vi "Convert Parameter string to 2D array.vi"(8 "Error In":errorcluster, 11 "Parameter string IN (without paranthesis)":string) -> (0 "Error Out":errorcluster, 1 "offset of last detected comma (0 if none)":i32, 2 "Number of commas":i32, 3 "Params table OUT":string[][](array[string]))   [LabVIEW 2012]
doc: "SciScan 1.2 160622"
uses:
  <vilib>/regexp/Match Regular Expression.xnode
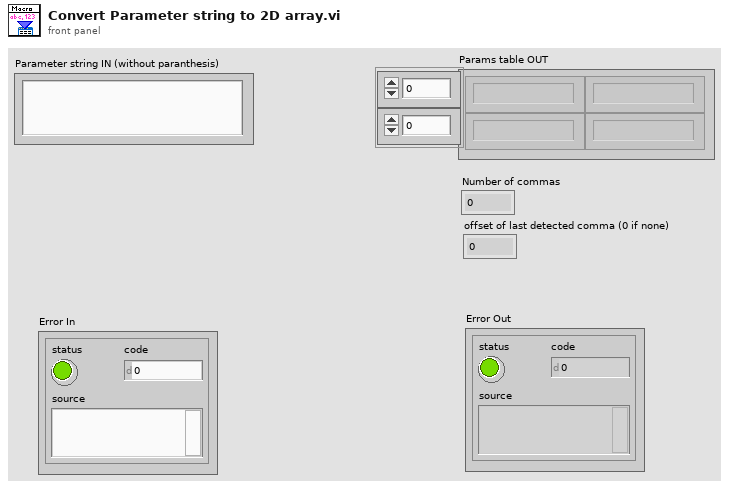
[diagram p1: front panel]
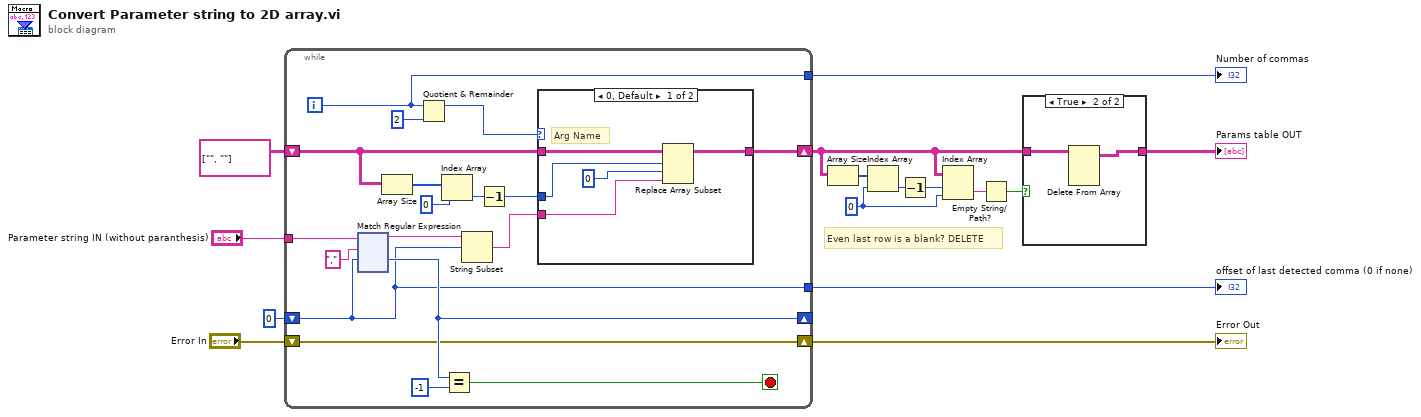
[diagram p0: block diagram]
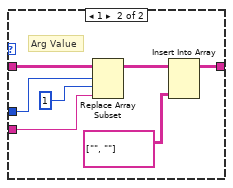
[diagram p3: hidden frame]
diagram:
  w3 = 0 ("index")
  # "Even last row is a blank? DELETE"
  n1 = while {
    tunnel: "Parameter string IN (without paranthesis)" -> [w32]
    shift-right: [w27] -> _
    shift-left: 0 ("offset past match") -> [w16]
    shift-right: [w22] -> w5
    shift-left: string[][] [["", ""]] -> [w19]
    shift-right: [w18] -> w12
    shift-left: "Error In" -> [w18]
    tunnel: [w17] -> w10
    tunnel: [w16] -> w9
    i -> [w17]
    stop <- w25 stop-if-true
    n2 = xnode "Match Regular Expression"("input string"=w32, "regular expression"="," ("search string/char (-)"), "offset (0)"=w16) -> ("before match"=w31:string, "offset past match"=w27:i32)  [unwired: 3 in, 3 out]
    n3 = Array Size(array=w19) -> (size(s)=w24:i32[])
    n4 = Quotient & Remainder(x=w17, y=2) -> (x-y*floor(x/y)=w29:i32)  [unwired: 1 out]
    n5 = Index Array(array=w24, index=0) -> (element=w21:i32)
    n6 = Equal?(x=w27, y=-1) -> (x = y?=w25:bool)
    n7 = String Subset(string=w31, offset (0)=w16) -> (substring=w28:string)  [unwired: 1 in]
    n8 = Decrement(x=w21) -> (x-1=w20:i32)
    n9 = case shown="0, Default" w29 {
      tunnel: w28 -> [w36 w42]
      tunnel: [w35 w39] -> w22
      tunnel: w19 -> [w37 w45]
      tunnel: w20 -> [w34 w44]
      frame 0, Default {
        # "Arg Name"
        n10 = Replace Array Subset(array=w37, new element=w36, index (row)=w34, index (col)=0 ("disabled index (col)")) -> (w35:string[][])
      }
      frame 1 {
        # "Arg Value"
        n11 = Replace Array Subset(array=w45, new element=w42, index (row)=w44, index (col)=1 ("disabled index (col)")) -> (w40:string[][])
        n12 = Insert Into Array(array=w40, new element=string[][] [["", ""]]) -> (w39:string[][])  [unwired: 2 in]
      }
    }
  }
  "Error Out" <- w12
  "Number of commas" <- w10
  "offset of last detected comma (0 if none)" <- w9
  n13 = Array Size(array=w5) -> (size(s)=w7:i32[])
  n14 = Index Array(array=w7, index=w3) -> (element=w6:i32)
  n15 = Decrement(x=w6) -> (x-1=w4:i32)
  n16 = Index Array(array=w5, index (row)=w4, index (col)=w3) -> (element=w2:string)
  n17 = Empty String/Path?(string/path=w2) -> (empty?=w1:bool)
  n18 = case shown="True" w1 {
    tunnel: [w157 w159] -> w8
    tunnel: w5 -> [w157 w158]
    frame False {
    }
    frame True {
      n19 = Delete From Array "Delete From Array"(array=w158) -> (array with subset deleted=w159:string[][])  [unwired: 3 in, 1 out]
    }
  }
  "Params table OUT" <- w8
